vi "Datasheet Single Item Generate.vi"(4 "Datasheets to Generate":T2[](array[typedef]), 5 "Grouped Results":cluster{"Result Group":T7[]}[](array[cluster]), 6 "Paths":T4[](array[typedef]), 7 "Generator Settings":T6={"Wait? (t)"=TRUE, "ClientPrint? (f)"=FALSE, "Client (\"\")"="", "joinPDF"=FALSE, "Sort Method"=enum."Item", "Export Row (-1=all)"=-1, "Preview"=FALSE, "Estimate Time"=FALSE, "username"="", "jobid"=""}, 8 "error in (no error)":errorcluster, 9 "Parameters":T3, 10 "Template Record":T5, 11 "Connection Refnum":T1) -> (0 "error out":errorcluster, 1 "Datasheets Generated":T2[](array[typedef]), 2 "Paths":T4[](array[typedef]), 3 "Connection Refnum":T1)   [LabVIEW 2011]
uses:
  Datasheet Report Info.ctl
  www/cgi-bin/_cgi-lib/TDM_INDEX Record.ctl
  Datasheet Generator Settings.ctl
  Summitek EXT/ODBC/SQL Controls/Connection Refnum.ctl
  database/Templates/Template Record.ctl
  ITK EXT/utils/keyedarr.llb/Keyed Array.ctl
  lib/datasheet script data.ctl
  database/Fields/Field Order By.ctl
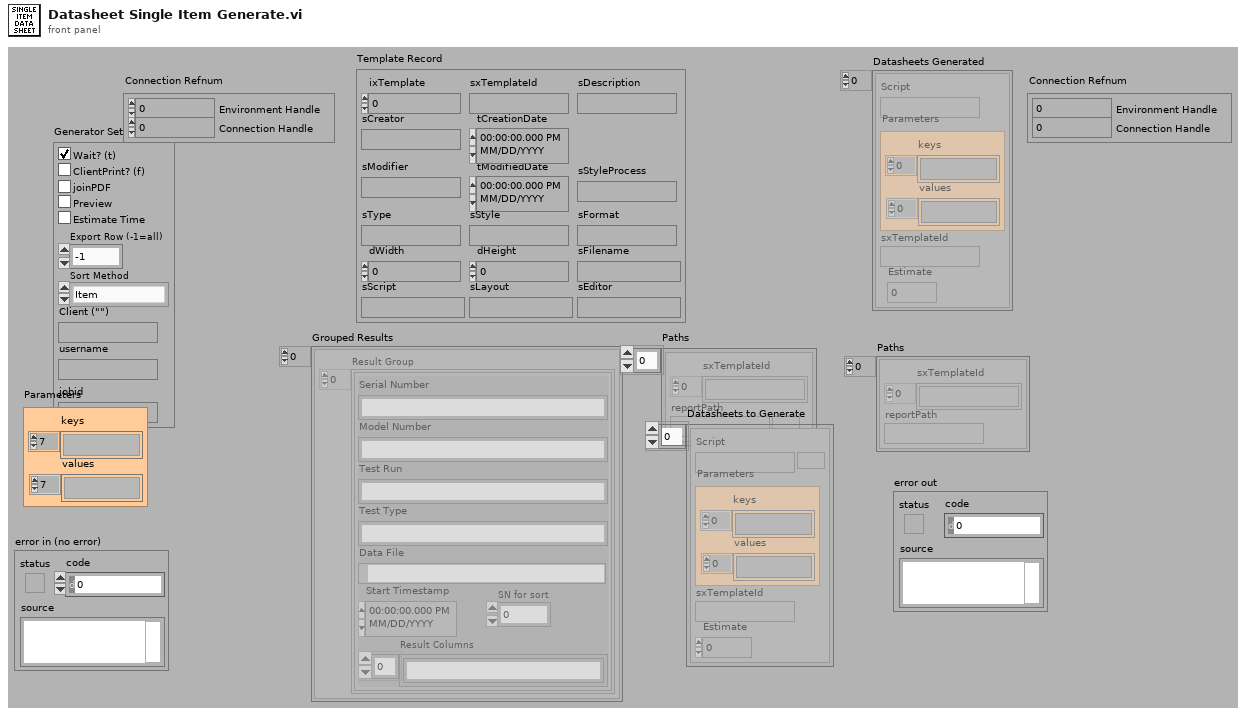
[diagram p1: front panel]
types:
  T1 = typedef "Connection Refnum.ctl" = cluster{"Environment Handle":i32, "Connection Handle":i32}
  T2 = typedef "datasheet script data.ctl" = cluster{"Script":path, "Parameters":T3, "sxTemplateId":string, "Estimate":i32}
  T3 = typedef "Keyed Array.ctl" = cluster{"keys":string[], "values":string[]}
  T4 = typedef "Datasheet Report Info.ctl" = cluster{"sxTemplateId":string[], "reportPath":path}
  T5 = typedef "Template Record.ctl" = cluster{"ixTemplate":i32, "sxTemplateId":string, "sDescription":string, "sCreator":string, "tCreationDate":timestamp, "sModifier":string, "tModifiedDate":timestamp, "sType":string, "sStyle":string, "sFormat":string, "dWidth":dbl, "dHeight":dbl, "sFilename":string, "sScript":string, "sLayout":string, "sEditor":string, "sStyleProcess":string}
  T6 = typedef "DATASHEET Generator Settings.ctl" = cluster{"Wait? (t)":bool, "ClientPrint? (f)":bool, "Client (\"\")":string, "joinPDF":bool, "Sort Method":enum16{"Item", "Template", "No Sort"}, "Export Row (-1=all)":i32, "Preview":bool, "Estimate Time":bool, "username":string, "jobid":string}
  T7 = typedef "TDM_INDEX Record.ctl" = cluster{"Model Number":string, "SN for sort":i32, "Test Type":string, "Test Run":string, "Serial Number":string, "Start Timestamp":timestamp, "Data File":path, "Result Columns":string[]}
  T8 = typedef "Field Order By.ctl" = enum32{"sxSequenceId", "sxFieldId", "sDisplayName", "sValue", "fSetAtTest", "fRequired", "nNextItem"}
  T9 = typedef "Field Record.ctl" = cluster{"ixField":i32, "iSequenceOrder":i32, "sxFieldId":string, "sxSequenceId":string, "sDisplayName":string, "sValue":string, "sUnits":string, "nDataType":T10, "nNextItem":T11, "fSystem":bool, "fSystemValue":bool, "fRequired":bool, "fSetAtTest":bool, "fTestField":bool, "fDeleted":bool, "fIndexed":bool, "fFreeList":bool}
  T10 = typedef "Field DataTypes.ctl" = enum32{"text", "numeric", "list", "timestamp", "boolean"}
  T11 = typedef "Field NextItem.ctl" = enum32{"Reset", "Retain", "Auto-Increment"}
  T12 = typedef "DATASHEET Field Display Names.ctl" = cluster{"Serial Number":string, "Model Number":string, "Sequence ID":string, "Start Time":string, "Instrument":string, "Company":string, "Operator":string, "test run":string}
  T13 = typedef "TDMS File.ctl" = cluster{"File Path":path, "Run Data":T14[], "Serial Number":string, "Model Number":string, "Test Type":string}
  T14 = typedef "TDMS Run.ctl" = cluster{"Channel Data":T15[], "Custom Fields":T9[], "Run ID":string}
  T15 = typedef "TDMS Channel (Sxx).ctl" = cluster{"Channel Name":string, "Waveform":dbl[], "Unit":string, "List value":string}
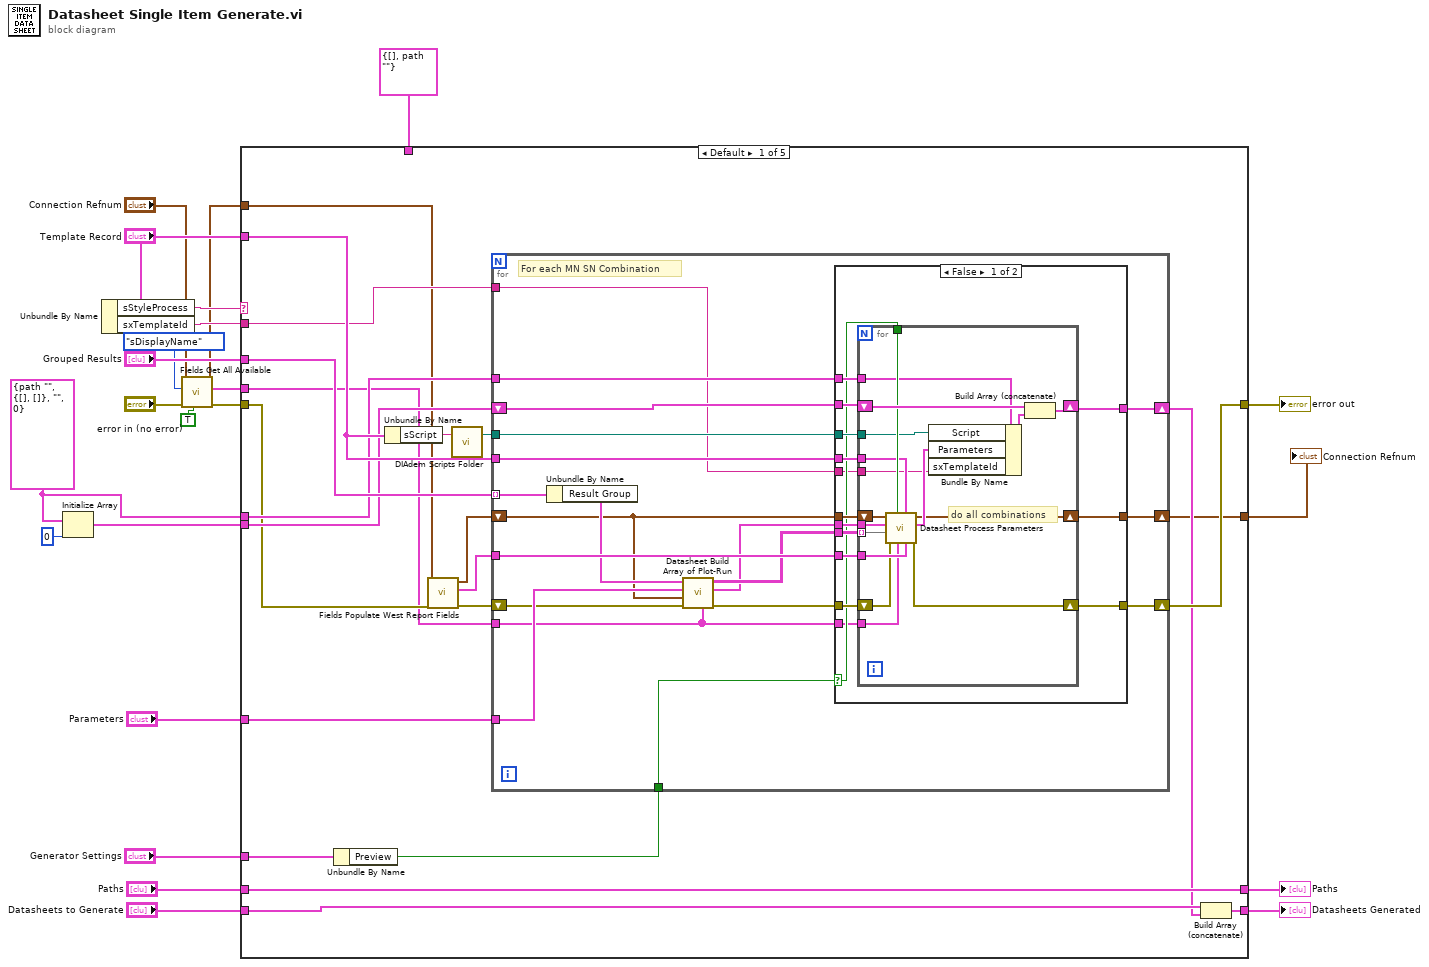
[diagram p0: block diagram]
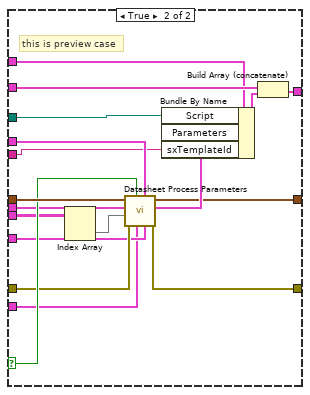
[diagram p2: hidden frame]
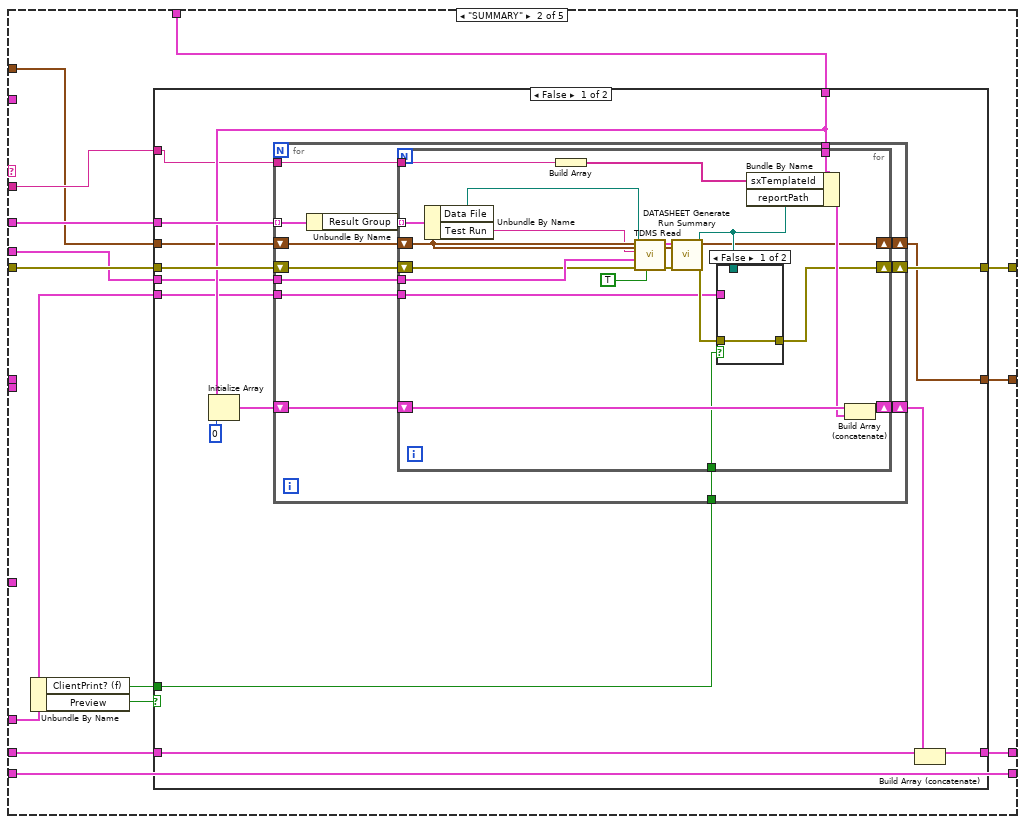
[diagram p3: hidden frame]
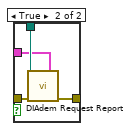
[diagram p4: hidden frame]
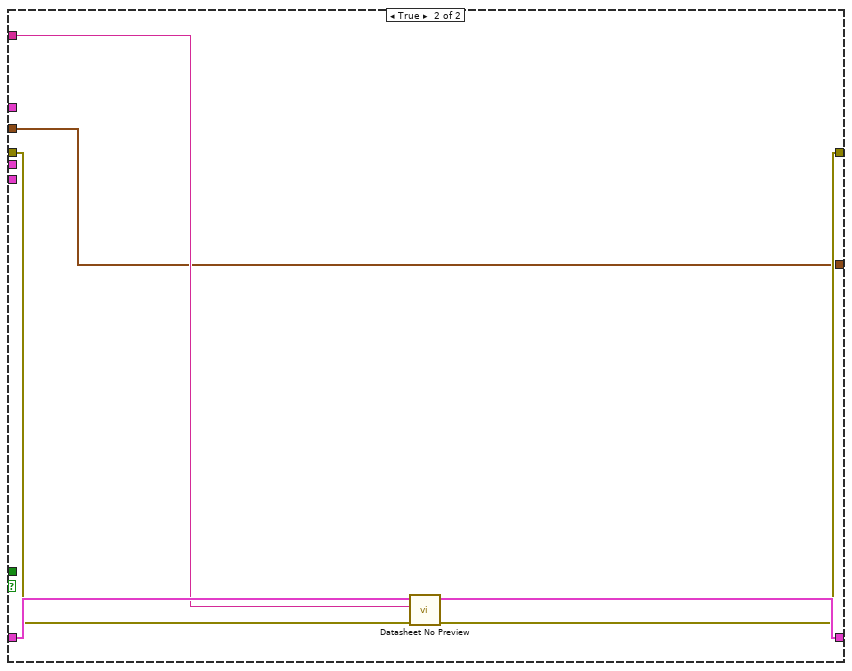
[diagram p5: hidden frame]
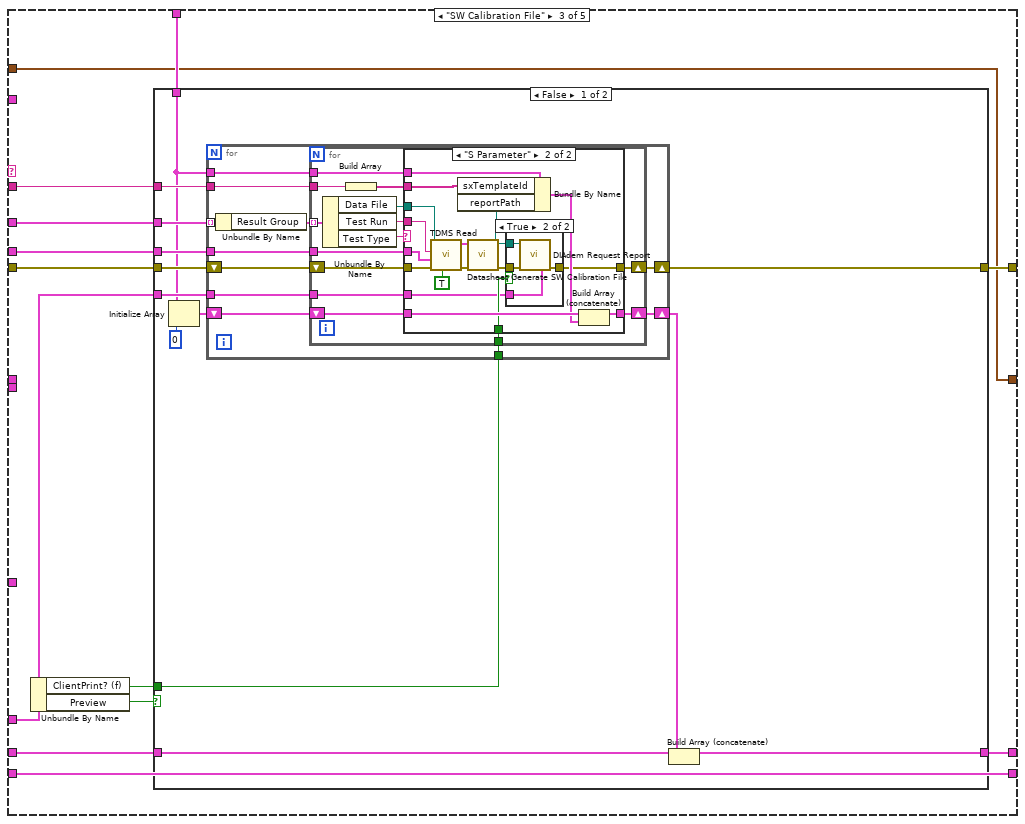
[diagram p6: hidden frame]
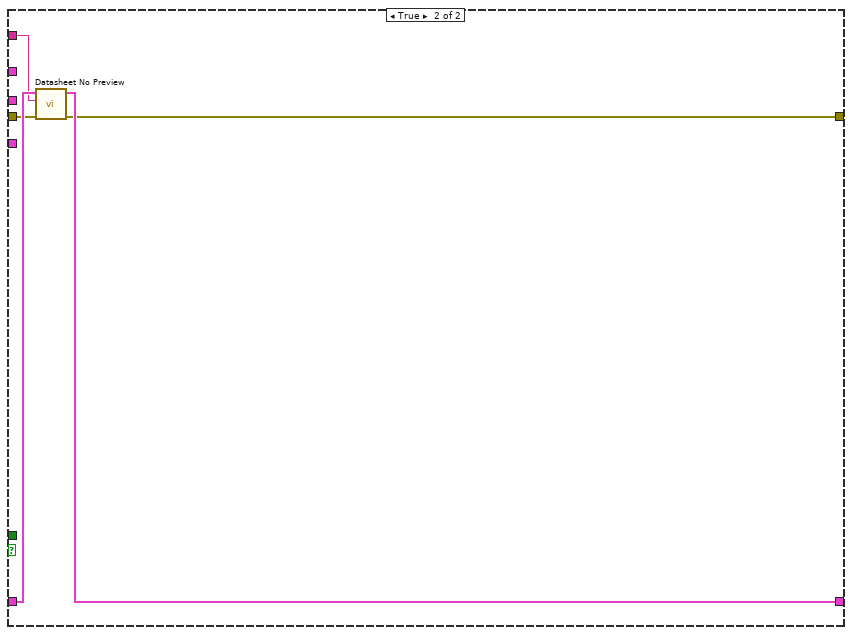
[diagram p9: hidden frame]
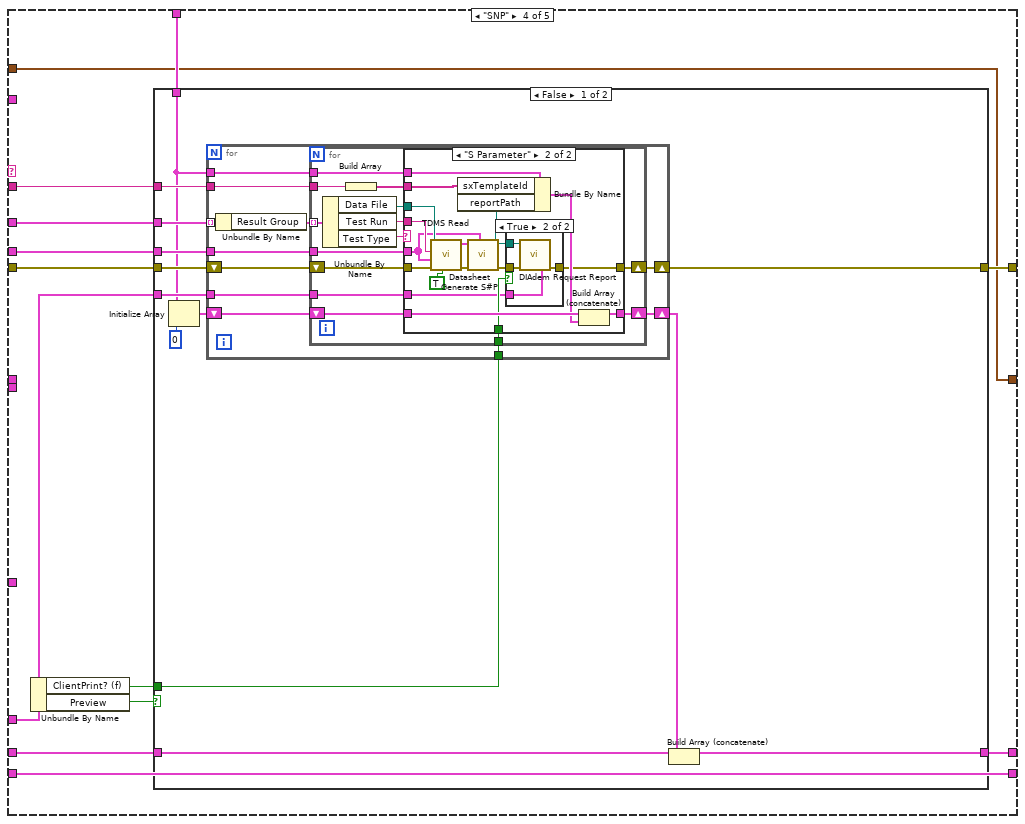
[diagram p10: hidden frame]
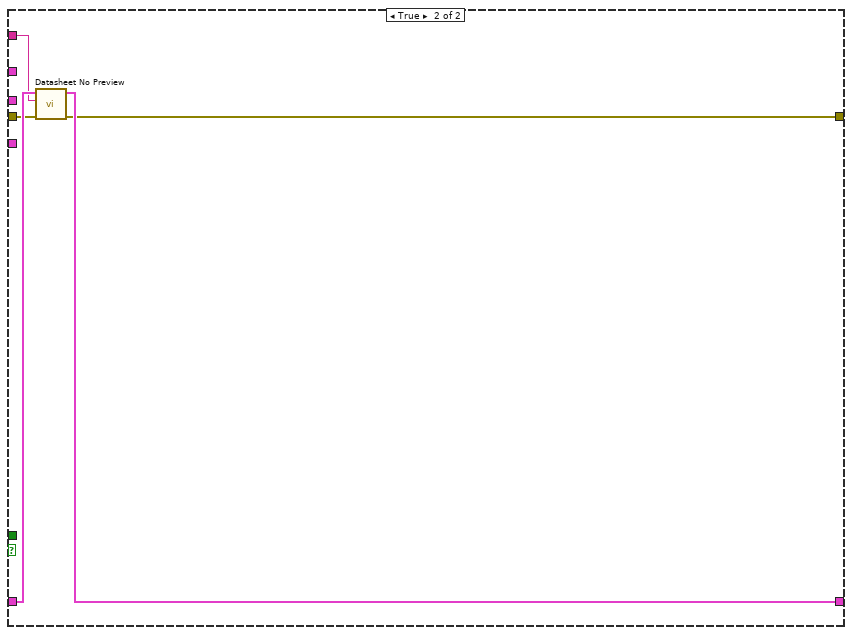
[diagram p13: hidden frame]
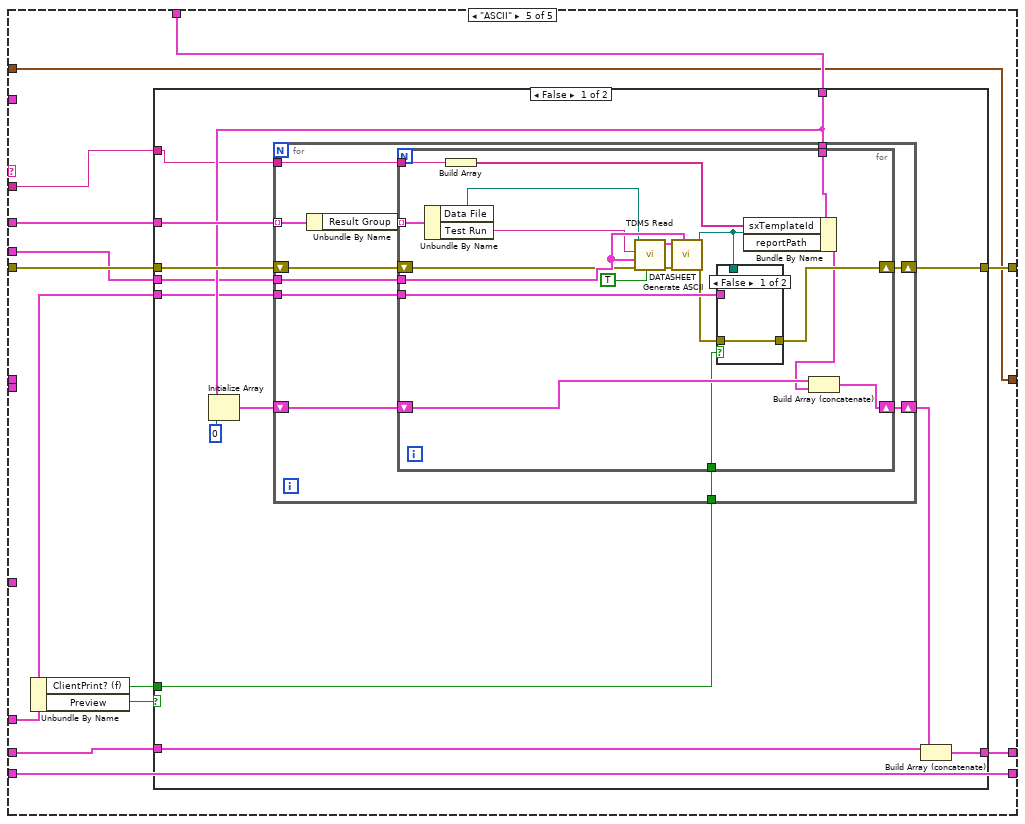
[diagram p14: hidden frame]
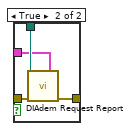
[diagram p15: hidden frame]
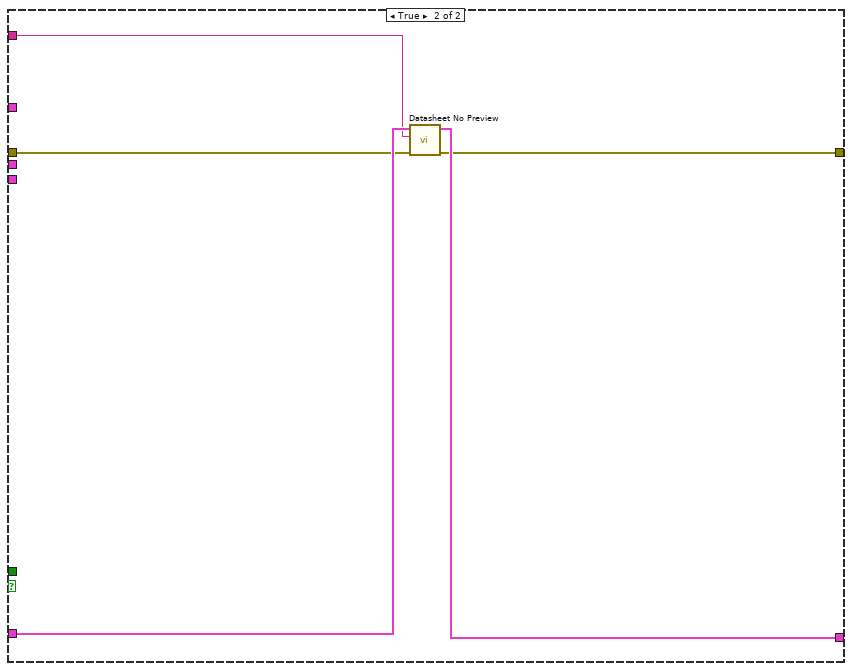
[diagram p16: hidden frame]
diagram:
  w13 = T2 {"Script"=path "", "Parameters"={"keys"=[], "values"=[]}, "sxTemplateId"="", "Estimate"=0} ("Datasheet")
  n1 = Initialize Array(w13, 0 ("dimension size")) -> (w14:T2[])
  n2 = Unbundle By Name("Template Record") -> ("sStyleProcess"=w19:string, "sxTemplateId"=w10:string)
  n3 = call "Fields Get All Available.vi"("Combine All? (f)"=TRUE, "error in (no error)"="error in (no error)", "Sort by (sxSequenceId)"=Field_Order_By."sDisplayName", "Connection Refnum"="Connection Refnum") -> ("error out"=w4:errorcluster, "System or ALL Combined Fields"=w1:T9[], "Connection Refnum"=w2:T1)  [unwired: 2 in, 3 out]
  n4 = case shown="Default" w19 {
    tunnel: [w34 w124 w196 w276 w356] -> w23
    tunnel: [w37 w128 w200 w280 w360] -> w22
    tunnel: w4 -> [w25 w116 w189 w268 w350]
    tunnel: "Grouped Results" -> [w43 w127 w199 w279 w359]
    tunnel: "Generator Settings" -> [w30 w119 w191 w271 w351]
    tunnel: w2 -> [w26 w117 w188 w270 w349]
    tunnel: "Template Record" -> [w42 _ _ _ _]
    tunnel: "Parameters" -> [w41 _ _ _ _]
    tunnel: [w33 w126 w198 w278 w358] -> w16
    tunnel: w14 -> [w39 _ _ _ _]
    tunnel: w13 -> [w38 _ _ _ _]
    tunnel: "Datasheets to Generate" -> [w32 w126 w198 w278 w358]
    tunnel: "Paths" -> [w34 w125 w197 w277 w357]
    tunnel: w10 -> [w28 w122 w194 w274 w354]
    tunnel: T4 {"sxTemplateId"=[], "reportPath"=path ""} ("report") -> [_ w121 w193 w273 w353]
    tunnel: [w27 w118 w188 w270 w349] -> w8
    tunnel: w1 -> [w24 w115 w190 w269 w348]
    frame Default {
      n5 = Unbundle By Name(w30) -> ("Preview"=w29:bool)
      n6 = Unbundle By Name(w42) -> ("sScript"=w40:string)
      n7 = call "Fields Populate West Report Fields.vi"("error in (no error)"=w25, "Connection Refnum"=w26) -> ("error out"=w44:errorcluster, "Report Field Display Names"=w45:T12, "Connection Refnum"=w36:T1)  [unwired: 1 in, 6 out]
      n8 = call "DIAdem Scripts Folder.vi"("Relative Path (\"\" - Folder)"=w40) -> ("Scripts Folder"=w35:path)  [unwired: 2 out]
      n9 = for {
        tunnel: w43 -> [w64] mode=indexing
        shift-right: [w61] -> w37
        shift-left: w44 -> [w54]
        shift-right: [w63] -> w31
        shift-left: w39 -> [w62]
        tunnel: w41 -> [w55]
        tunnel: w45 -> [w60]
        tunnel: w42 -> [w59]
        tunnel: w38 -> [w58]
        tunnel: w35 -> [w57]
        tunnel: w29 -> [w51]
        tunnel: w28 -> [w50]
        tunnel: w24 -> [w47]
        shift-right: [w46] -> w27
        shift-left: w36 -> [w48]
        # "For each MN SN Combination"
        n10 = Unbundle By Name(w64) -> ("Result Group"=w56:T7[])
        n11 = call "Datasheet Build Array of Plot-Run.vi"("System or ALL Combined Fields"=w47, "error in (no error)"=w54, "Connection Refnum"=w48, "Parameters"=w55, "Result Group"=w56) -> ("error out"=w53:errorcluster, "Updated Parameter"=w49:T3, "Runs for Each Plot"=w52:T13[][])  [unwired: 1 in, 3 out]
        n12 = case shown="False" w51 {
          selector: w51 -> [w68 w113]
          tunnel: [w79 w104] -> w63
          tunnel: w62 -> [w78 w105]
          tunnel: [w77 w110] -> w61
          tunnel: w60 -> [w76 w109]
          tunnel: w48 -> [w75 w114]
          tunnel: w59 -> [w74 w102]
          tunnel: w58 -> [w73 w103]
          tunnel: w57 -> [w72 w107]
          tunnel: w49 -> [w71 w112]
          tunnel: w53 -> [w70 w111]
          tunnel: w52 -> [w69 w101]
          tunnel: w50 -> [w67 w99]
          tunnel: w47 -> [w66 w98]
          tunnel: [w65 w97] -> w46
          frame False {
            n13 = for {
              tunnel: w76 -> [w93]
              tunnel: w68 -> [w90]
              tunnel: w71 -> [w89]
              shift-right: [w96] -> w79
              shift-left: w78 -> [w95]
              shift-right: [w94] -> w77
              shift-left: w70 -> [w91]
              tunnel: w74 -> [w88]
              tunnel: w72 -> [w86]
              tunnel: w73 -> [w85]
              tunnel: w69 -> [w84] mode=indexing
              tunnel: w67 -> [w80]
              tunnel: w66 -> [w82]
              shift-right: [w81] -> w65
              shift-left: w75 -> [w92]
              # "do all combinations"
              n14 = call "Datasheet Process Parameters.vi"("Report Field Display Names"=w93, "Template Record"=w88, "System or ALL Combined Fields"=w82, "Preview?"=w90, "error in (no error)"=w91, "Runs for this plot"=w84, "Parameters"=w89, "Connection Refnum"=w92) -> ("error out"=w94:errorcluster, "Parameters"=w87:T3, "Connection Refnum"=w81:T1)  [unwired: 1 in]
              n15 = Bundle By Name(cluster=w85, "Script"=w86, "Parameters"=w87, "sxTemplateId"=w80) -> (w83:T2)
              n16 = Build Array (concatenate)(w95, w83) -> (w96:T2[])
            }
          }
          frame True {
            # "this is preview case"
            n17 = Index Array(array=w101) -> (element=w100:T13[])  [unwired: 2 in]
            n18 = call "Datasheet Process Parameters.vi"("Report Field Display Names"=w109, "Template Record"=w102, "System or ALL Combined Fields"=w98, "Preview?"=w113, "error in (no error)"=w111, "Runs for this plot"=w100, "Parameters"=w112, "Connection Refnum"=w114) -> ("error out"=w110:errorcluster, "Parameters"=w106:T3, "Connection Refnum"=w97:T1)  [unwired: 1 in]
            n19 = Bundle By Name(cluster=w103, "Script"=w107, "Parameters"=w106, "sxTemplateId"=w99) -> (w108:T2)
            n20 = Build Array (concatenate)(w105, w108) -> (w104:T2[])
          }
        }
      }
      n21 = Build Array (concatenate)(w32, w31) -> (w33:T2[])
    }
    frame "SUMMARY" {
      n22 = Unbundle By Name(w119) -> ("ClientPrint? (f)"=w120:bool, "Preview"=w123:bool)
      n23 = case shown="False" w123 {
        tunnel: [w143 w184] -> w128
        tunnel: w127 -> [w142 _]
        tunnel: w116 -> [w141 w185]
        tunnel: w125 -> [w140 w187]
        tunnel: [w139 w186] -> w124
        tunnel: w122 -> [w137 w183]
        tunnel: w121 -> [w138 _]
        tunnel: w120 -> [w136 _]
        tunnel: w119 -> [w135 _]
        tunnel: w115 -> [w134 _]
        tunnel: w117 -> [w130 w182]
        tunnel: [w129 w182] -> w118
        frame False {
          n24 = Initialize Array(w138, 0 ("dimension size")) -> (w133:T4[])
          n25 = for {
            tunnel: w142 -> [w151] mode=indexing
            shift-right: [w152] -> w131
            shift-left: w133 -> [w153]
            shift-right: [w154] -> w143
            shift-left: w141 -> [w155]
            tunnel: w138 -> [w150]
            tunnel: w137 -> [w149]
            tunnel: w136 -> [w148]
            tunnel: w135 -> [w147]
            tunnel: w134 -> [w146]
            shift-right: [w144] -> w129
            shift-left: w130 -> [w145]
            n26 = Unbundle By Name(w151) -> ("Result Group"=w156:T7[])
            n27 = for {
              tunnel: w156 -> [w176] mode=indexing
              shift-right: [w174] -> w152
              shift-left: w153 -> [w175]
              shift-right: [w163] -> w154
              shift-left: w155 -> [w159]
              tunnel: w150 -> [w170]
              tunnel: w149 -> [w168]
              tunnel: w148 -> [w166]
              tunnel: w147 -> [w162]
              tunnel: w146 -> [w161]
              shift-right: [w160] -> w144
              shift-left: w145 -> [w160]
              n28 = Unbundle By Name(w176) -> ("Data File"=w157:path, "Test Run"=w158:string)
              n29 = Build Array(w168) -> (w167:string[])
              n30 = call "TDMS Read.vi"("Load Fields?"=TRUE, "error in (no error)"=w159, "System or ALL Combined Fields"=w161, "Run String"=w158, "TDM File Path"=w157) -> ("error out"=w172:errorcluster, "File Information"=w173:T13)  [unwired: 2 in, 3 out]
              n31 = call "DATASHEET Generate Run Summary.vi"("Connection Refnum"=w160, "error in (no error)"=w172, "File Information"=w173) -> ("error out"=w164:errorcluster, "Summary File Path"=w165:path)  [unwired: 1 in, 6 out]
              n32 = case shown="False" w166 {
                tunnel: w165 -> [_ w181]
                tunnel: w164 -> [w177 w180]
                tunnel: [w177 w179] -> w163
                tunnel: w162 -> [_ w178]
                frame False {
                }
                frame True {
                  n33 = call "DIAdem Request Report.vi"("Report Path\n(empty - auto PDF in user's folder)"=w181, "generator settings"=w178, "error in (no error)"=w180) -> ("error out"=w179:errorcluster)  [unwired: 12 out]
                }
              }
              n34 = Bundle By Name(cluster=w170, "sxTemplateId"=w167, "reportPath"=w165) -> (w169:T4)
              n35 = Build Array (concatenate)(w175, w169) -> (w174:T4[])
            }
          }
          n36 = Build Array (concatenate)(w140, w131) -> (w139:T4[])
        }
        frame True {
          n37 = call "Datasheet No Preview.vi"("error in"=w185, "sxTemplateId"=w183, "Paths"=w187) -> ("error out"=w184:errorcluster, "Array"=w186:T4[])  [unwired: 7 out]
        }
      }
    }
    frame "SW Calibration File" {
      n38 = Unbundle By Name(w191) -> ("ClientPrint? (f)"=w192:bool, "Preview"=w195:bool)
      n39 = case shown="False" w195 {
        tunnel: [w213 w264] -> w200
        tunnel: w199 -> [w212 _]
        tunnel: w189 -> [w211 w265]
        tunnel: w197 -> [w210 w267]
        tunnel: [w209 w266] -> w196
        tunnel: w194 -> [w208 w263]
        tunnel: w193 -> [w201 _]
        tunnel: w192 -> [w207 _]
        tunnel: w191 -> [w206 _]
        tunnel: w190 -> [w202 _]
        frame False {
          n40 = Initialize Array(w201, 0 ("dimension size")) -> (w205:T4[])
          n41 = for {
            tunnel: w212 -> [w219] mode=indexing
            shift-right: [w220] -> w203
            shift-left: w205 -> [w221]
            shift-right: [w222] -> w213
            shift-left: w211 -> [w223]
            tunnel: w208 -> [w218]
            tunnel: w207 -> [w217]
            tunnel: w206 -> [w216]
            tunnel: w202 -> [w215]
            tunnel: w201 -> [w214]
            n42 = Unbundle By Name(w219) -> ("Result Group"=w224:T7[])
            n43 = for {
              tunnel: w224 -> [w238] mode=indexing
              shift-right: [w236] -> w220
              shift-left: w221 -> [w237]
              shift-right: [w232] -> w222
              shift-left: w223 -> [w235]
              tunnel: w218 -> [w234]
              tunnel: w217 -> [w233]
              tunnel: w216 -> [w231]
              tunnel: w215 -> [w227]
              tunnel: w214 -> [w225]
              n44 = Unbundle By Name(w238) -> ("Data File"=w228:path, "Test Run"=w230:string, "Test Type"=w226:string)
              n45 = Build Array(w234) -> (w229:string[])
              n46 = case shown="\"S Parameter\"" w226 {
                tunnel: w237 -> [w239 w257]
                tunnel: [w239 w256] -> w236
                tunnel: w230 -> [_ w247]
                tunnel: w235 -> [w240 w248]
                tunnel: w233 -> [_ w251]
                tunnel: [w240 w249] -> w232
                tunnel: w231 -> [_ w246]
                tunnel: w229 -> [_ w244]
                tunnel: w228 -> [_ w243]
                tunnel: w227 -> [_ w242]
                tunnel: w225 -> [_ w241]
                frame Default {
                }
                frame "S Parameter" {
                  n47 = call "TDMS Read.vi"("Load Fields?"=TRUE, "error in (no error)"=w248, "System or ALL Combined Fields"=w242, "Run String"=w247, "TDM File Path"=w243) -> ("error out"=w254:errorcluster, "File Information"=w255:T13)  [unwired: 2 in, 3 out]
                  n48 = call "Datasheet Generate SW Calibration File.vi"("error in (no error)"=w254, "File Information"=w255) -> ("error out"=w250:errorcluster, "SW Cal File Path"=w245:path)  [unwired: 8 in]
                  n49 = Bundle By Name(cluster=w241, "sxTemplateId"=w244, "reportPath"=w245) -> (w252:T4)
                  n50 = case shown="True" w251 {
                    tunnel: w250 -> [w258 w262]
                    tunnel: [w258 w261] -> w249
                    tunnel: w246 -> [_ w260]
                    tunnel: w245 -> [_ w259]
                    frame False {
                    }
                    frame True {
                      n51 = call "DIAdem Request Report.vi"("Report Path\n(empty - auto PDF in user's folder)"=w259, "generator settings"=w260, "error in (no error)"=w262) -> ("error out"=w261:errorcluster)  [unwired: 12 out]
                    }
                  }
                  n52 = Build Array (concatenate)(w257, w252) -> (w256:T4[])
                }
              }
            }
          }
          n53 = Build Array (concatenate)(w210, w203) -> (w209:T4[])
        }
        frame True {
          n54 = call "Datasheet No Preview.vi"("error in"=w265, "sxTemplateId"=w263, "Paths"=w267) -> ("error out"=w264:errorcluster, "Array"=w266:T4[])  [unwired: 7 out]
        }
      }
    }
    frame "SNP" {
      n55 = Unbundle By Name(w271) -> ("ClientPrint? (f)"=w272:bool, "Preview"=w275:bool)
      n56 = case shown="False" w275 {
        tunnel: [w293 w344] -> w280
        tunnel: w279 -> [w292 _]
        tunnel: w268 -> [w291 w345]
        tunnel: w277 -> [w290 w347]
        tunnel: [w289 w346] -> w276
        tunnel: w274 -> [w288 w343]
        tunnel: w273 -> [w281 _]
        tunnel: w272 -> [w287 _]
        tunnel: w271 -> [w286 _]
        tunnel: w269 -> [w282 _]
        frame False {
          n57 = Initialize Array(w281, 0 ("dimension size")) -> (w285:T4[])
          n58 = for {
            tunnel: w292 -> [w299] mode=indexing
            shift-right: [w300] -> w283
            shift-left: w285 -> [w301]
            shift-right: [w302] -> w293
            shift-left: w291 -> [w303]
            tunnel: w288 -> [w298]
            tunnel: w287 -> [w297]
            tunnel: w286 -> [w296]
            tunnel: w282 -> [w295]
            tunnel: w281 -> [w294]
            n59 = Unbundle By Name(w299) -> ("Result Group"=w304:T7[])
            n60 = for {
              tunnel: w304 -> [w318] mode=indexing
              shift-right: [w316] -> w300
              shift-left: w301 -> [w317]
              shift-right: [w312] -> w302
              shift-left: w303 -> [w315]
              tunnel: w298 -> [w314]
              tunnel: w297 -> [w313]
              tunnel: w296 -> [w311]
              tunnel: w295 -> [w307]
              tunnel: w294 -> [w305]
              n61 = Unbundle By Name(w318) -> ("Data File"=w308:path, "Test Run"=w310:string, "Test Type"=w306:string)
              n62 = Build Array(w314) -> (w309:string[])
              n63 = case shown="\"S Parameter\"" w306 {
                tunnel: w317 -> [w319 w337]
                tunnel: [w319 w336] -> w316
                tunnel: w310 -> [_ w327]
                tunnel: w315 -> [w320 w328]
                tunnel: w313 -> [_ w331]
                tunnel: [w320 w329] -> w312
                tunnel: w311 -> [_ w326]
                tunnel: w309 -> [_ w324]
                tunnel: w308 -> [_ w323]
                tunnel: w307 -> [_ w322]
                tunnel: w305 -> [_ w321]
                frame Default {
                }
                frame "S Parameter" {
                  n64 = call "TDMS Read.vi"("Load Fields?"=TRUE, "error in (no error)"=w328, "System or ALL Combined Fields"=w322, "Run String"=w327, "TDM File Path"=w323) -> ("error out"=w334:errorcluster, "File Information"=w335:T13)  [unwired: 2 in, 3 out]
                  n65 = call "Datasheet Generate S#P.vi"("System or ALL Combined Fields"=w322, "error in (no error)"=w334, "File Information"=w335) -> ("error out"=w330:errorcluster, "SNP File Path"=w325:path)  [unwired: 7 in]
                  n66 = Bundle By Name(cluster=w321, "sxTemplateId"=w324, "reportPath"=w325) -> (w332:T4)
                  n67 = case shown="True" w331 {
                    tunnel: w330 -> [w338 w342]
                    tunnel: [w338 w341] -> w329
                    tunnel: w326 -> [_ w340]
                    tunnel: w325 -> [_ w339]
                    frame False {
                    }
                    frame True {
                      n68 = call "DIAdem Request Report.vi"("Report Path\n(empty - auto PDF in user's folder)"=w339, "generator settings"=w340, "error in (no error)"=w342) -> ("error out"=w341:errorcluster)  [unwired: 12 out]
                    }
                  }
                  n69 = Build Array (concatenate)(w337, w332) -> (w336:T4[])
                }
              }
            }
          }
          n70 = Build Array (concatenate)(w290, w283) -> (w289:T4[])
        }
        frame True {
          n71 = call "Datasheet No Preview.vi"("error in"=w345, "sxTemplateId"=w343, "Paths"=w347) -> ("error out"=w344:errorcluster, "Array"=w346:T4[])  [unwired: 7 out]
        }
      }
    }
    frame "ASCII" {
      n72 = Unbundle By Name(w351) -> ("ClientPrint? (f)"=w352:bool, "Preview"=w355:bool)
      n73 = case shown="False" w355 {
        tunnel: [w373 w410] -> w360
        tunnel: w359 -> [w372 _]
        tunnel: w350 -> [w371 w411]
        tunnel: w357 -> [w370 w413]
        tunnel: [w369 w412] -> w356
        tunnel: w354 -> [w367 w409]
        tunnel: w353 -> [w368 _]
        tunnel: w352 -> [w366 _]
        tunnel: w351 -> [w365 _]
        tunnel: w348 -> [w364 _]
        frame False {
          n74 = Initialize Array(w368, 0 ("dimension size")) -> (w363:T4[])
          n75 = for {
            tunnel: w372 -> [w379] mode=indexing
            shift-right: [w380] -> w361
            shift-left: w363 -> [w381]
            shift-right: [w382] -> w373
            shift-left: w371 -> [w383]
            tunnel: w368 -> [w378]
            tunnel: w367 -> [w377]
            tunnel: w366 -> [w376]
            tunnel: w365 -> [w375]
            tunnel: w364 -> [w374]
            n76 = Unbundle By Name(w379) -> ("Result Group"=w384:T7[])
            n77 = for {
              tunnel: w384 -> [w403] mode=indexing
              shift-right: [w401] -> w380
              shift-left: w381 -> [w402]
              shift-right: [w396] -> w382
              shift-left: w383 -> [w385]
              tunnel: w378 -> [w400]
              tunnel: w377 -> [w399]
              tunnel: w376 -> [w397]
              tunnel: w375 -> [w395]
              tunnel: w374 -> [w394]
              n78 = Unbundle By Name(w403) -> ("Data File"=w386:path, "Test Run"=w387:string)
              n79 = Build Array(w399) -> (w398:string[])
              n80 = call "TDMS Read.vi"("Load Fields?"=TRUE, "error in (no error)"=w385, "System or ALL Combined Fields"=w394, "Run String"=w387, "TDM File Path"=w386) -> ("error out"=w392:errorcluster, "File Information"=w393:T13)  [unwired: 2 in, 3 out]
              n81 = call "DATASHEET Generate ASCII.vi"("System or ALL Combined Fields"=w394, "error in (no error)"=w392, "File Information"=w393) -> ("error out"=w388:errorcluster, "ASCII File Path"=w389:path)  [unwired: 7 in]
              n82 = case shown="False" w397 {
                tunnel: w389 -> [_ w408]
                tunnel: w388 -> [w404 w407]
                tunnel: [w404 w406] -> w396
                tunnel: w395 -> [_ w405]
                frame False {
                }
                frame True {
                  n83 = call "DIAdem Request Report.vi"("Report Path\n(empty - auto PDF in user's folder)"=w408, "generator settings"=w405, "error in (no error)"=w407) -> ("error out"=w406:errorcluster)  [unwired: 12 out]
                }
              }
              n84 = Bundle By Name(cluster=w400, "sxTemplateId"=w398, "reportPath"=w389) -> (w390:T4)
              n85 = Build Array (concatenate)(w402, w390) -> (w401:T4[])
            }
          }
          n86 = Build Array (concatenate)(w370, w361) -> (w369:T4[])
        }
        frame True {
          n87 = call "Datasheet No Preview.vi"("error in"=w411, "sxTemplateId"=w409, "Paths"=w413) -> ("error out"=w410:errorcluster, "Array"=w412:T4[])  [unwired: 7 out]
        }
      }
    }
  }
  "Paths" <- w23
  "error out" <- w22
  "Datasheets Generated" <- w16
  "Connection Refnum" <- w8
